vi "MTM2_putSample_temperature.vi"(8 "error in (no error)":errorcluster, 11 "temperature_Ctl":T1={"private_rcvStamp"=0.0, "ring[12]"=[0.0, 0.0, 0.0, 0.0, 0.0, 0.0, 0.0, 0.0, 0.0, 0.0, 0.0, 0.0], "intake[2]"=[0.0, 0.0], "exhaust[2]"=[0.0, 0.0]}) -> (0 "error out":errorcluster, 2 "function return":i32, 3 "temperature_Ctl out":T1)   [LabVIEW 2018, in "SALLV_MTM2.lvlib"]
doc: "int MTM2_shm_putSample_temperatureLV(MTM2_temperatureLV *temperature_Ctl );"
uses:
  DataTypes/temperature.ctl
  SALLV_MTM2.lvlib
  SALLV_MTM2.so
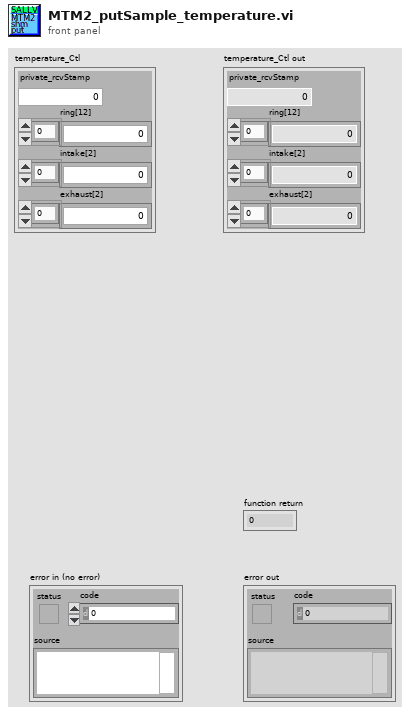
[diagram p1: front panel]
types:
  T1 = typedef "SALLV_MTM2.lvlib/temperature.ctl" = cluster{"private_rcvStamp":dbl, "ring[12]":dbl[], "intake[2]":dbl[], "exhaust[2]":dbl[]}
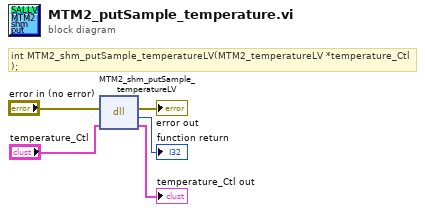
[diagram p0: block diagram]
diagram:
  # "int MTM2_shm_putSample_temperatureLV(MTM2_temperatureLV *temperature_Ctl );"
  n1 = dll-call lib="home/ttsai/Documents/salLabviewApi/SALLV_MTM2/SALLV_MTM2.*" fn="MTM2_shm_putSample_temperatureLV"(error in="error in (no error)", "temperature_Ctl"="temperature_Ctl") -> (error out=→"error out":errorcluster, →"function return":i32, "temperature_Ctl"=→"temperature_Ctl out":T1)  [unwired: 2 in, 1 out]
